vi "arrayEqual00000sfp+.vi"(3 "input_array":u8[](array[numeric])) -> (1 "show_bool_result":bool)   [LabVIEW 2011]
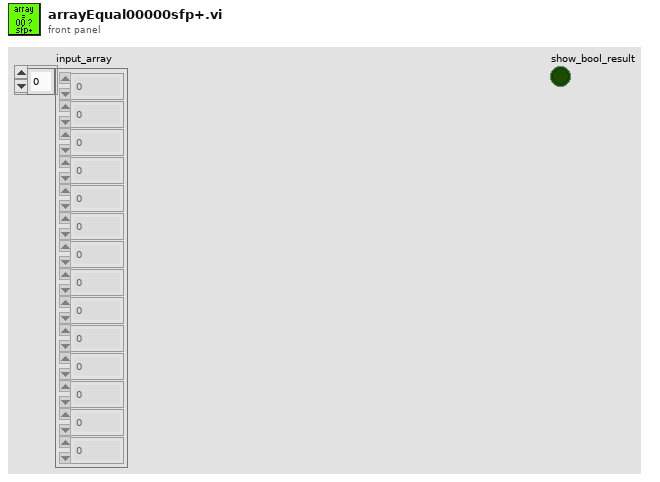
[diagram p1: front panel]
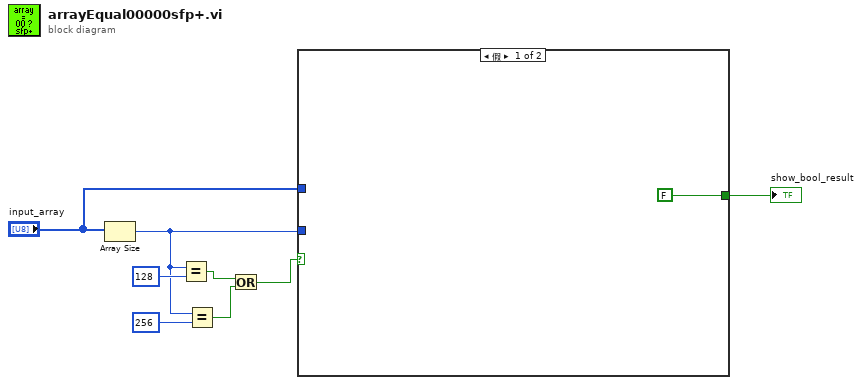
[diagram p0: block diagram]
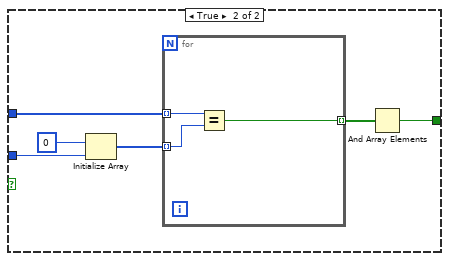
[diagram p2: hidden frame]
diagram:
  n1 = Array Size(array="input_array") -> (size(s)=w6:i32)
  n2 = Equal?(x=w6, y=128) -> (x = y?=w5:bool)
  n3 = Equal?(x=w6, y=256) -> (x = y?=w4:bool)
  n4 = Or(x=w5, y=w4) -> (x .or. y?=w3:bool)
  n5 = case shown="假" w3 {
    tunnel: w6 -> [_ w14]
    tunnel: "input_array" -> [_ w13]
    tunnel: [FALSE w10] -> w1
    frame False {
    }
    frame True {
      n6 = Initialize Array(u8 0, w14) -> (w12:u8[])
      n7 = for {
        tunnel: w13 -> [w18] mode=indexing
        tunnel: w12 -> [w17] mode=indexing
        tunnel: [w16] -> w11 mode=indexing
        n8 = Equal?(x=w18, y=w17) -> (x = y?=w16:bool)
      }
      n9 = And Array Elements(Boolean array=w11) -> (logical AND=w10:bool)
    }
  }
  "show_bool_result" <- w1
